vi "Set Pulse Repetition Frequency [PRF].vi"(7 "Micropulse # In":i32, 8 "error in (no error)":errorcluster, 10 "Frequency (Hz)":u16) -> (0 "error out":errorcluster, 5 "Micropulse # Out":i32)   [LabVIEW 2026, in "MicroPulse_Driver.lvlib"]
doc: "The <rate> parameter specifies the maximum rate in firings per second. The time period is derived from a timer device and so is accurate provided that the rate specified is not greater than that which MicroPulse can achieve or the ultrasonics will allow.\n\nParameters:\n<rate> : Test repetition rate in Hz, between 1 Hz and 20 kHz in 1 Hz steps.\n\nExample:\nPRF 1000 \nSets PRF. of 1000 Hz. This ensures that firings will be at least 1 millisecond apart."
uses:
  MicroPulse_Driver.lvlib
  Private/MP-Registry Action-Enum.ctl
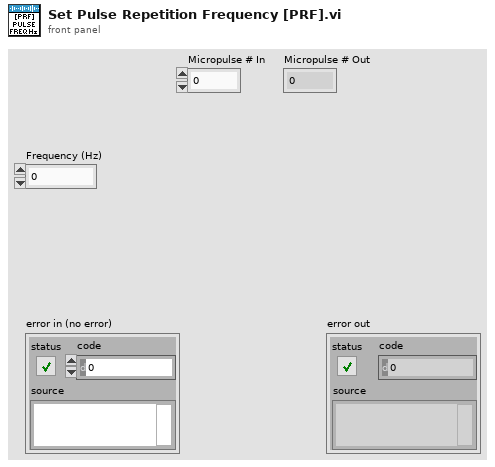
[diagram p1: front panel]
types:
  T1 = typedef "MicroPulse_Driver.lvlib/MP-Registry Action-Enum.ctl" = enum16{"Read", "Add Test", "Add Command", "Add Gate Command", "Add Encoder Command", "Clear Command  List", "Set Registry", "Set System Details", "Set DOF", "Set Velocity", "Disable Asynch Reads", "Enable Asynch Reads", "Add Connection", "Disconnect", "Shutdown"}
  T2 = typedef "MicroPulse_Driver.lvlib/TCP config.ctl" = cluster{"Connection ID":refnum<k5>, "IP address":string, "host port":u16, "OC timeout":i32, "Read timeout":i32, "Write timeout":i32}
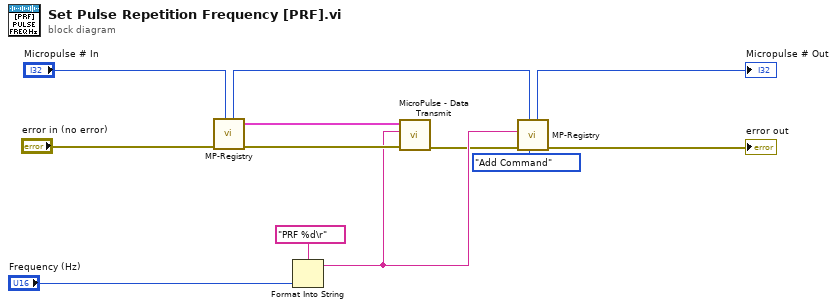
[diagram p0: block diagram]
diagram:
  n1 = call "MP-Registry.vi"("Micropulse # In"="Micropulse # In", "error in (no error)"="error in (no error)") -> ("error out"=w10:errorcluster, "TCP config"=w9:T2, "Micropulse # Out"=w5:i32)  [unwired: 6 in, 1 out]
  n2 = Format Into String(format string="PRF %d\r", "Frequency (Hz)") -> (resulting string=w8:string)  [unwired: 2 in, 1 out]
  n3 = call "MicroPulse - Data Transmit.vi"("error in (no error)"=w10, "data"=w8, "TCP config"=w9) -> ("error out"=w6:errorcluster)  [unwired: 6 in, 2 out]
  n4 = call "MP-Registry.vi"("Action"=MP-Registry_Action-Enum."Add Command", "Micropulse # In"=w5, "error in (no error)"=w6, "Data in"=w8) -> ("error out"=→"error out":errorcluster, "Micropulse # Out"=→"Micropulse # Out":i32)  [unwired: 4 in, 2 out]
